vi "dfd_PR Cosine-Modulated Rotate.vi"(11 "angle":dbl) -> (3 "rotate":dbl[][](array[numeric]))   [LabVIEW 2017, in "NI_DigFilter_FilterBank.lvlib"]
uses:
  <vilib>/addons/Digital Filter Design/NI_DigFilter_FilterBank.lvlib
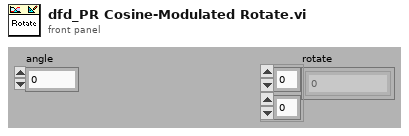
[diagram p1: front panel]
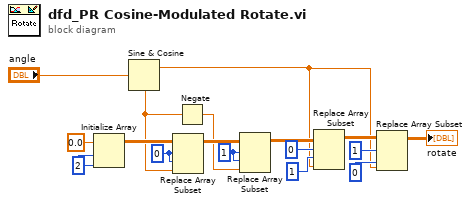
[diagram p0: block diagram]
diagram:
  w11 = 1 ("index (row)")
  w14 = 0 ("index (row)")
  w16 = 2
  n1 = Initialize Array(0.0 ("element"), w16, w16) -> (w15:dbl[][])
  n2 = Sine & Cosine(0:"angle") -> (1:w3:dbl, 2:w13:dbl)
  n3 = Replace Array Subset(array=w15, new element=w13, index (row)=w14, index (col)=w14) -> (w12:dbl[][])
  n4 = Negate(x=w13) -> (-x=w10:dbl)
  n5 = Replace Array Subset(array=w12, new element=w10, index (row)=w11, index (col)=w11) -> (w7:dbl[][])
  n6 = Replace Array Subset(array=w7, new element=w3, index (row)=0, index (col)=1 ("disabled index (col)")) -> (w6:dbl[][])
  n7 = Replace Array Subset(array=w6, new element=w3, index (row)=1, index (col)=0 ("disabled index (col)")) -> (→"rotate":dbl[][])
